vi "(SubVI) ignore the row contain zero from 2D array.vi"(11 "Array in":dbl[][](array[numeric])) -> (3 "Array out":dbl[][](array[numeric]))   [LabVIEW 2016]
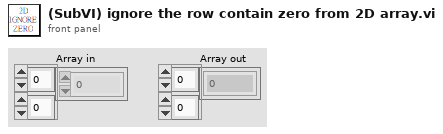
[diagram p1: front panel]
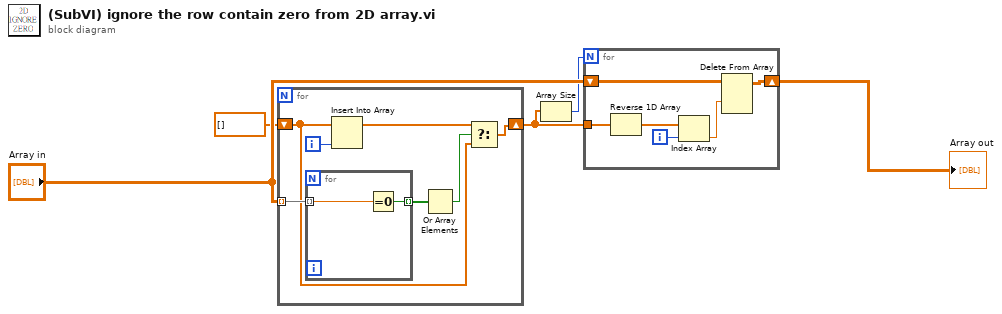
[diagram p0: block diagram]
diagram:
  n1 = for {
    tunnel: "Array in" -> [w12] mode=indexing
    shift-right: [w6] -> w3
    shift-left: dbl[] [] -> [w9]
    i -> [w10]
    n2 = for {
      tunnel: w12 -> [w14] mode=indexing
      tunnel: [w13] -> w11 mode=indexing
      n3 = Equal To 0?(x=w14) -> (x = 0?=w13:bool)
    }
    n4 = Insert Into Array(array=w9, new element=w10) -> (w8:dbl[])  [unwired: 1 in]
    n5 = Or Array Elements(Boolean array=w11) -> (logical OR=w7:bool)
    n6 = Select(t=w8, s=w7, f=w9) -> (s? t:f=w6:dbl[])
  }
  n7 = Array Size(array=w3) -> (size(s)=w2:i32)
  n8 = for {
    N: w2 -> [_]
    tunnel: w3 -> [w20]
    shift-right: [w18] -> w5
    shift-left: "Array in" -> [w19]
    i -> [w16]
    n9 = Reverse 1D Array(array=w20) -> (reversed array=w17:dbl[])
    n10 = Index Array(array=w17, index=w16) -> (element=w15:dbl)
    n11 = Delete From Array(array=w19, index (row)=w15) -> (array with subset deleted=w18:dbl[][])  [unwired: 2 in, 1 out]
  }
  "Array out" <- w5
